vi "joystick control MS3.vi"() -> ()   [LabVIEW 2014]
uses:
  <vilib>/Utility/inputDevices.llb/joystickAcquire.vi
  <vilib>/Utility/inputDevices.llb/closeJoystick.vi
panel:
  out "direction info":T1
  out "button info":T2
  in  "stop 2":bool
  in  "device index":i32
  out "joystick info":T3(array[cluster])
  out "Z axis":i32
  out "Y axis":i32
  out "X axis":i32
  out "error out":errorcluster
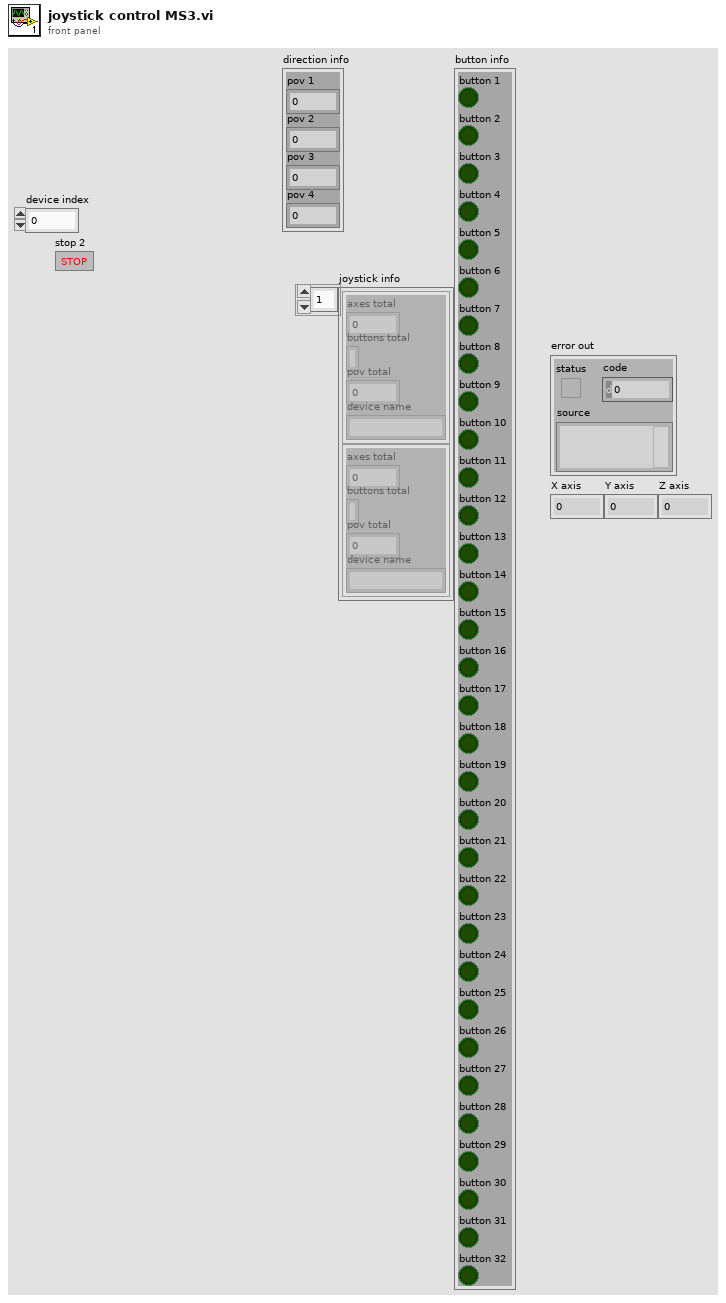
[diagram p1: front panel]
types:
  T1 = cluster{"pov 1":i32, "pov 2":i32, "pov 3":i32, "pov 4":i32}
  T2 = cluster{"button 1":bool, "button 2":bool, "button 3":bool, "button 4":bool, "button 5":bool, "button 6":bool, "button 7":bool, "button 8":bool, "button 9":bool, "button 10":bool, "button 11":bool, "button 12":bool, "button 13":bool, "button 14":bool, "button 15":bool, "button 16":bool, "button 17":bool, "button 18":bool, "button 19":bool, "button 20":bool, "button 21":bool, "button 22":bool, "button 23":bool, "button 24":bool, "button 25":bool, "button 26":bool, "button 27":bool, "button 28":bool, "button 29":bool, "button 30":bool, "button 31":bool, "button 32":bool}
  T3 = cluster{"axes total":u32, "buttons total":u32, "pov total":u32, "device name":string}[]
  T4 = cluster{"X axis":i32, "Y axis":i32, "Z axis":i32, "X axis rotation":i32, "Y axis rotation":i32, "Z axis rotation":i32, "U axis":i32, "V axis":i32}
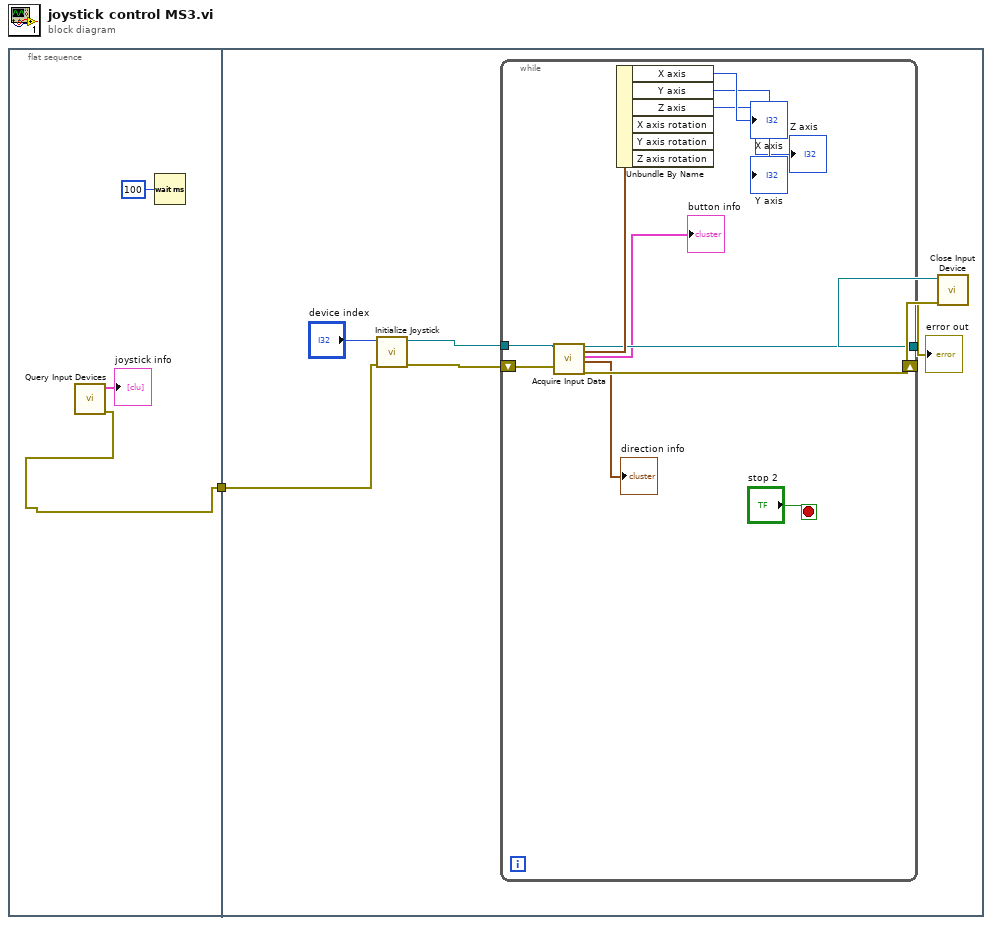
[diagram p0: block diagram]
diagram:
  n1 = flat-sequence {
    tunnel: [w3] -> w1
    tunnel: w1 -> [w5]
    frame #0 {
      n2 = call <vilib>:"Query Input Devices.vi"() -> ("error out"=w3:errorcluster, "joystick info"=→"joystick info":T3)  [unwired: 8 in, 2 out]
      n3 = Wait (ms)(milliseconds to wait=u32 100) -> ()  [unwired: 1 out]
    }
    frame #1 {
      n4 = call <vilib>:"Initialize Joystick.vi"("error in (no error)"=w5, "device index"="device index") -> ("error out"=w10:errorcluster, "device ID"=w9:refnum<k1>)  [unwired: 8 in]
      n5 = while {
        tunnel: w9 -> [w22]
        shift-right: [w15] -> w8
        shift-left: w10 -> [w20]
        tunnel: [w14] -> w6
        stop <- "stop 2" stop-if-true
        n6 = call-poly <vilib>:"Acquire Input Data.vi"("device ID"=w22, "error in (no error)"=w20) -> ("device ID 2"=w14:refnum<k1>, "axis info"=w21:T4, "button info"=→"button info":T2, "direction info"=→"direction info":T1, "error out"=w15:errorcluster)  [unwired: 13 in]
        n7 = Unbundle By Name(w21) -> ("X axis"=→"X axis":i32, "Y axis"=→"Y axis":i32, "Z axis"=→"Z axis":i32)  [unwired: 3 out]
      }
      n8 = call-poly <vilib>:"Close Input Device.vi"("error in (no error)"=w8, "device ID"=w6) -> ("error out"=→"error out":errorcluster)  [unwired: 8 in]
    }
  }
